vi "select_waveforms.vi"(0 "Trace controls":T6[](array[typedef]), 5 "Flag selectors":T4[](array[typedef]), 9 "Pose selectors":T1[](array[typedef]), 11 "Decimate":i32=1, 12 "Reference hold":bool) -> (4 "Waveforms out":waveform(sgl)[](array[waveform]), 6 "Digital waveforms":digitalwaveform[](array[waveform]), 8 "XY views":cluster{"X":sgl[], "Y":sgl[]}[](array[cluster]), 15 "New data":bool)   [LabVIEW 2013]
uses:
  Trace controls.ctl
  probe_point.ctl
  flag_selector.ctl
  status_flag.ctl
  pose_selector.ctl
  pose_source.ctl
  pose_relative_to.ctl
panel:
  out "Reference":sgl[][](array[numeric])
  out "Last waveforms out":waveform(sgl)[](array[waveform])
  in  "Old trace counter":u32
  # "Locals"
  # "Trace record that is the base for relative display"
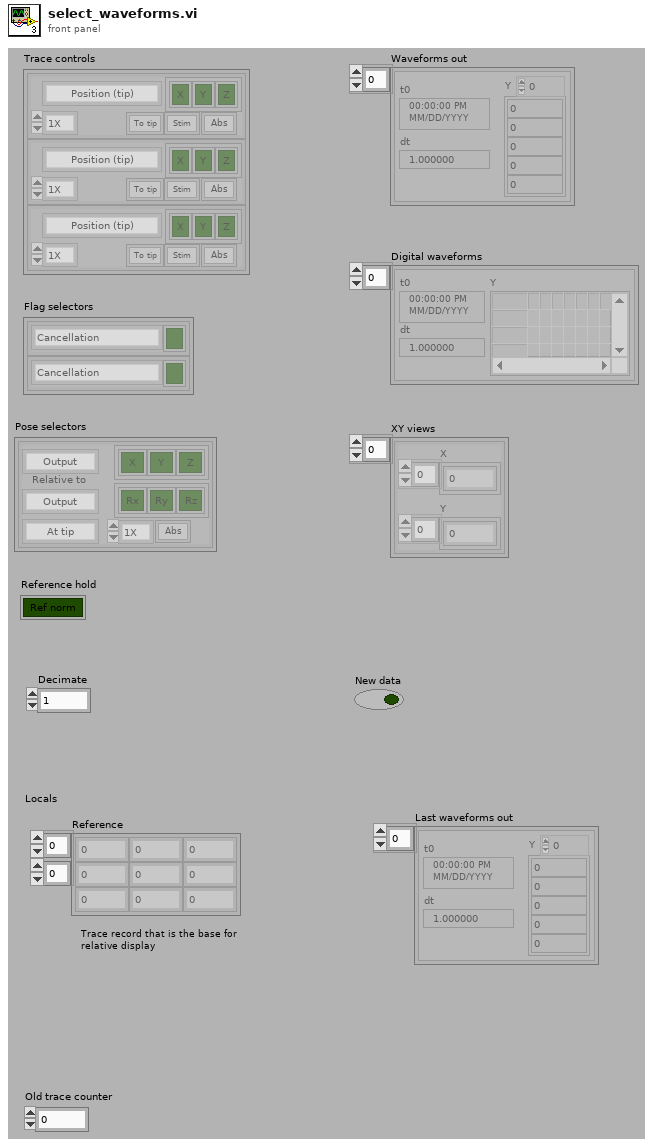
[diagram p1: front panel]
types:
  T1 = typedef "pose_selector.ctl" = cluster{"Scale":enum16{"1X", "10X", "100X", "1KX", "10KX"}, "Source":T2, "XYZ selector":cluster{"Boolean":bool, "Boolean 2":bool, "Boolean 3":bool}, "RPY selector":cluster{"Boolean":bool, "Boolean 2":bool, "Boolean 3":bool}, "Relative to":T3, "Relative":bool, "Translate":enum16{"At tip", "At RCM", "At KC", "At origin"}}
  T2 = typedef "pose_source.ctl" = enum16{"Output", "Handle", "Handle KF", "Goal", "Absolute"}
  T3 = typedef "pose_relative_to.ctl" = enum16{"Output", "Handle", "Handle KF", "Goal", "Absolute", "Trace start"}
  T4 = typedef "flag_selector.ctl" = cluster{"Flag":T5, "Select":bool}
  T5 = typedef "status_flag.ctl" = enum16{"Cancellation", "Goal filter", "Valid position", "Goal saturation tip", "Goal saturation RCM", "Goal circle saturation", "Position saturation", "Output saturation", "Acceleration limiting", "Finished late", "Stimulus increasing", "Integral error saturation", "Velocity limiting", "Log warning", "Log error", "Link KF degraded"}
  T6 = typedef "Trace controls.ctl" = cluster{"+ stim":bool, "Relative":bool, "Scale":enum16{"1X", "10X", "100X", "1KX", "10KX"}, "Probe point":T7, "XYZ selector":cluster{"Boolean":bool, "Boolean 2":bool, "Boolean 3":bool}, "To tip":bool}
  T7 = typedef "probe_point.ctl" = enum16{"Position (tip)", "Position (RCM)", "Null pos (tip)", "Null pos (RCM)", "V limiter (tip)", "V Limiter (RCM)", "Goal (tip)", "Goal (RCM)", "Link pos 0", "Link pos 1", "KF link pos 0", "KF link pos 1", "Link rate 0", "Link rate 1", "Link residue 0", "Link residue 1", "Link goal 0", "Link goal 1", "Rate limit 0", "Rate limit 1", "Link error 0", "Link error 1", "Controller 0", "Controller 1", "Output 0", "Output 1", "Drive 0", "Drive 1", "Stimulus 0", "Stimulus 1", "Trace data 0", "Trace data 1", "Analog data 0", "Analog data 1", "Status flags", "Light 0", "Light 1", "Light 2", "Light 3", "Light 4", "Light 5", "Goal origin", "Goal rotation 0", "Goal rotation 1", "Goal rotation 2", "Output origin", "Output rotation 0", "Output rotation 1", "Output rotation 2", "Handle origin", "Handle rotation 0", "Handle rotation 1", "Handle rotation 2", "Handle position", "Handle velocity", "Handle acceleration", "Handle angles", "Handle angle rates", "Handle pos residue", "Handle angle residue", "Trace length"}
  T8 = cluster{"Trace controls":T6[], "Flag selectors":T4[], "Decimate":i32, "Pose selectors":T1[], "Reference hold":bool}
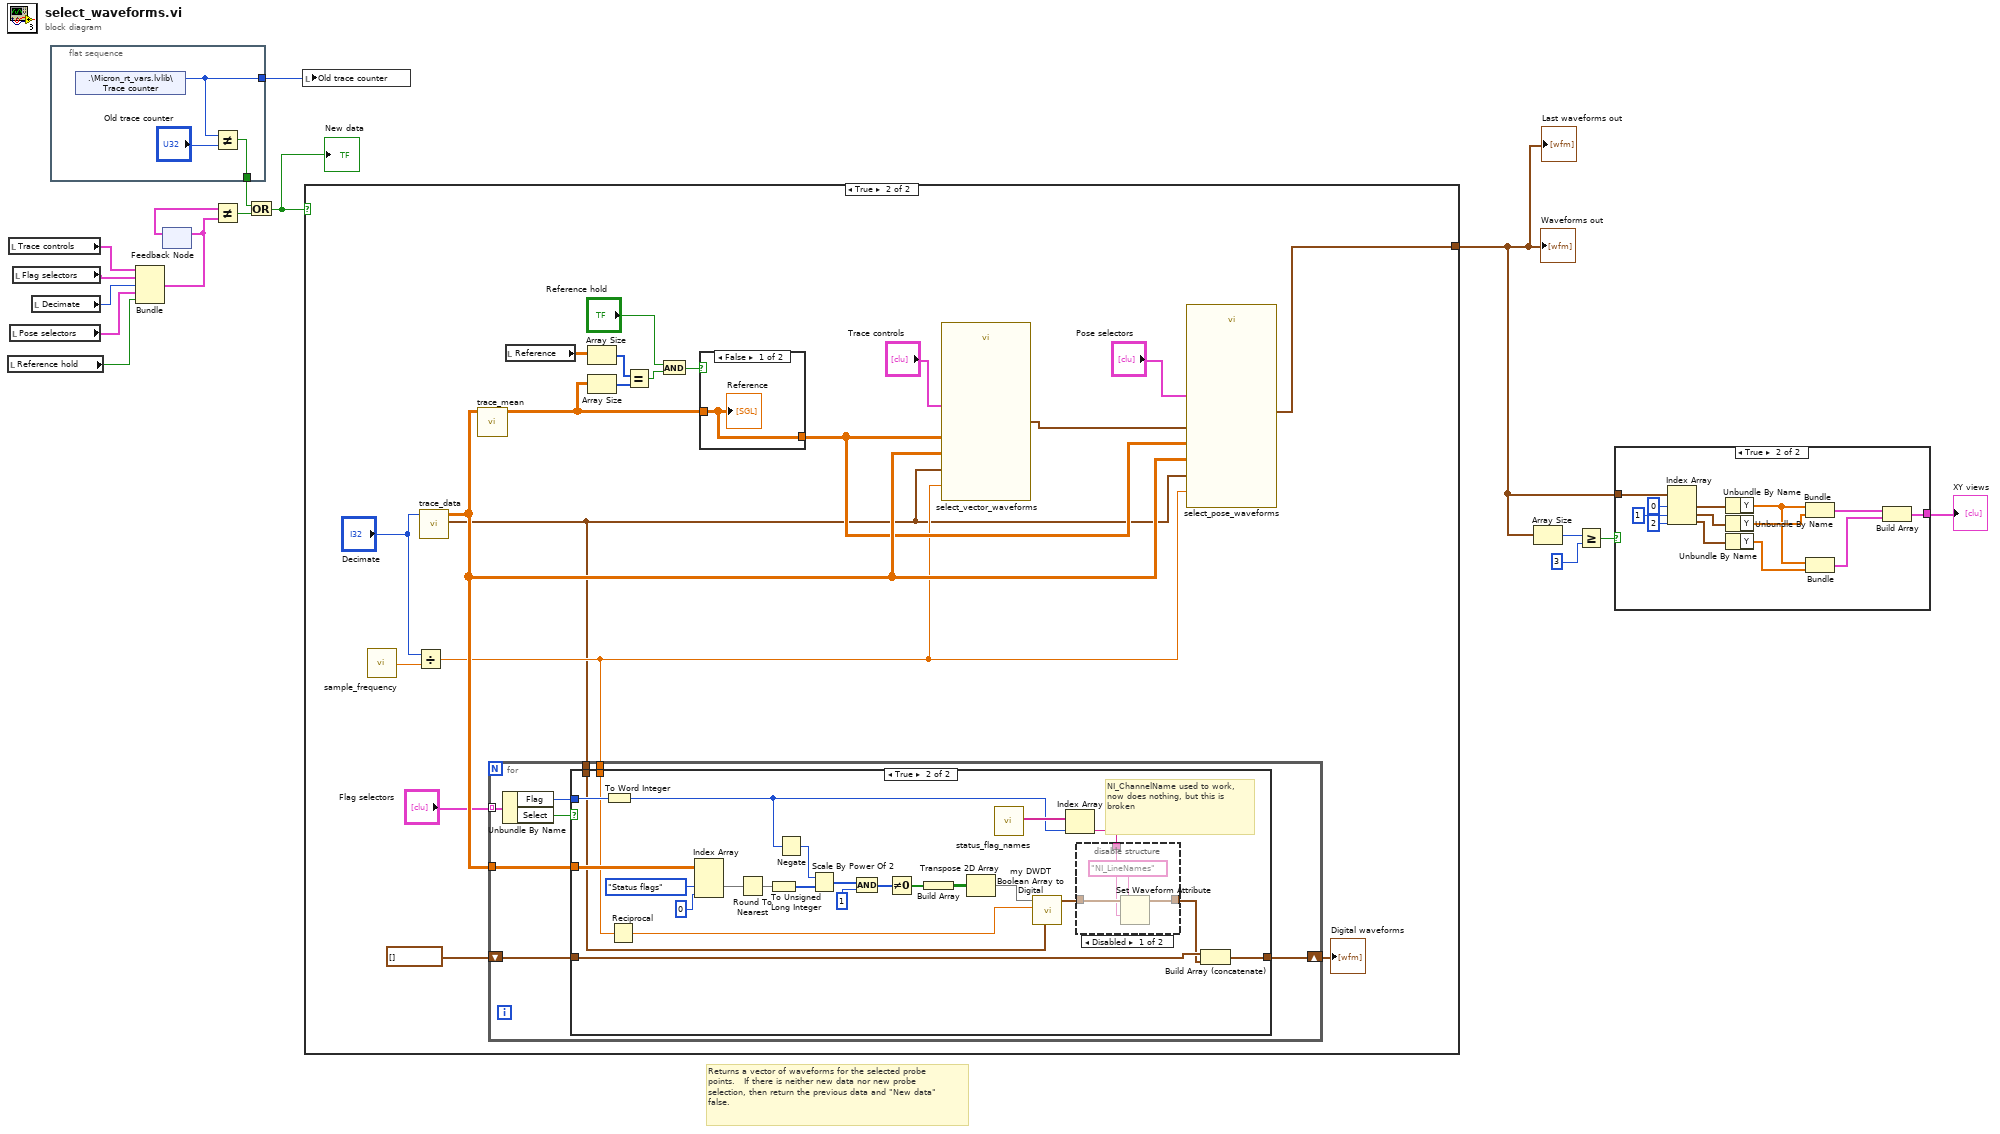
[diagram p0: block diagram]
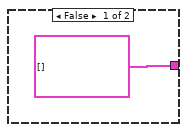
[diagram p2: hidden frame]
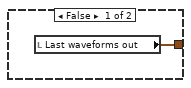
[diagram p3: hidden frame]
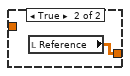
[diagram p4: hidden frame]
diagram:
  # "Returns a vector of waveforms for the selected probe points.   If there is neither new data nor new probe selection, then return the previous data and \"New data\" false."
  n1 = local read "Reference hold"() -> (w2:bool)
  n2 = local read "Trace controls"() -> (w8:T6[])
  n3 = local read "Pose selectors"() -> (w5:T1[])
  n4 = local read "Flag selectors"() -> (w7:T4[])
  n5 = local read "Decimate"() -> (w6:i32)
  n6 = flat-sequence {
    tunnel: [w18] -> w11
    tunnel: [w17] -> w16
    frame #0 {
      n7 = shared-variable ".\\Micron_rt_vars.lvlib\\Trace counter"() -> (w17:u32)  [unwired: 2 out]
      n8 = Not Equal?(x=w17, y="Old trace counter") -> (x != y?=w18:bool)
    }
  }
  n9 = Bundle("Trace controls"=w8, "Flag selectors"=w7, "Decimate"=w6, "Pose selectors"=w5, "Reference hold"=w2) -> (w4:T8)  [unwired: 1 in]
  n10 = feedback-in #1(w4) -> ()
  n11 = feedback #1() -> (w3:T8)  [unwired: 1 in]
  n12 = Not Equal?(x=w3, y=w4) -> (x != y?=w10:bool)
  n13 = Or(x=w11, y=w10) -> (x .or. y?=w9:bool)
  "New data" <- w9
  n14 = local write "Old trace counter"(w16) -> ()
  n15 = case shown="True" w9 {
    tunnel: [w20 w26] -> w1
    frame False {
      n16 = local read "Last waveforms out"() -> (w20:waveform(sgl)[])
    }
    frame True {
      n17 = call "sample_frequency.vi"() -> ("Sample frequency"=w39:dbl)
      n18 = Divide(x="Decimate", y=w39) -> (x/y=w23:dbl)
      n19 = call "trace_data.vi"("Decimate"="Decimate") -> ("Trace timestamp"=w21:timestamp, "Decimated trace"=w40:sgl[][][])  [unwired: 8 in, 1 out]
      n20 = call "trace_mean.vi"("Array in"=w40) -> ("Array out"=w22:sgl[][])  [unwired: 10 in]
      n21 = for {
        tunnel: "Flag selectors" -> [w50] mode=indexing
        tunnel: w40 -> [w48]
        shift-right: [w45] -> w35
        shift-left: digitalwaveform[] [] -> [w46]
        tunnel: w23 -> [w44]
        tunnel: w21 -> [w43]
        n22 = Unbundle By Name(w50) -> ("Flag"=w47:T5, "Select"=w49:bool)
        n23 = case shown="True" w49 {
          tunnel: w48 -> [_ w75]
          tunnel: w47 -> [_ w70]
          tunnel: w46 -> [w51 w64]
          tunnel: [w51 w60] -> w45
          tunnel: w44 -> [_ w62]
          tunnel: w43 -> [_ w53]
          frame False {
          }
          frame True {
            # "NI_ChannelName used to work, now does nothing, but this is broken"
            n24 = To Word Integer(number=w70) -> (16bit integer=w57:i16)
            n25 = Reciprocal(x=w62) -> (1/x=w61:dbl)
            n26 = Index Array(array=w75, index (dim 1)=probe_point."Status flags" ("Probe point"), index (dim 2)=0 ("disabled index (col)")) -> (element=w72:sgl[])  [unwired: 1 in]
            n27 = Round To Nearest(number=w72) -> (nearest integer value=w71:sgl[])
            n28 = To Unsigned Long Integer(number=w71) -> (unsigned 32bit integer=w68:u32[])
            n29 = Negate(x=w57) -> (-x=w69:i16)
            n30 = Scale By Power Of 2(n=w69, x=w68) -> (x*2^n=w67:u32[])
            n31 = And(x=w67, y=u32 1 ("disabled index (col)")) -> (x .and. y?=w65:u32[])
            n32 = Not Equal To 0?(x=w65) -> (x != 0?=w63:bool[])
            n33 = Build Array(w63) -> (w55:bool[][])
            n34 = Transpose 2D Array(2D array=w55) -> (transposed array=w54:bool[][])
            n35 = call "status_flag_names.vi"() -> ("Names"=w58:string[])  [unwired: 11 in]
            n36 = call "my DWDT Boolean Array to Digital.vi"("t0"=w53, "sample rate"=w61, "boolean array"=w54) -> ("digital waveform"=w59:digitalwaveform)  [unwired: 7 in, 1 out]
            n37 = Index Array(array=w58, index=w57) -> (element=w56:string)
            n38 = disable-structure shown="Disabled" {
              disable-tunnel: w59 -> [w78 w80]
              disable-tunnel: w56 -> [w77 _]
              disable-tunnel: [w76 w80] -> w52
              frame Disabled {
                n39 = Set Waveform Attribute(5:w77, 6:"NI_LineNames" ("name"), 7:w78) -> (3:w76:digitalwaveform)  [unwired: 1 in, 2 out]
              }
              frame Enabled {
              }
            }
            n40 = Build Array (concatenate)(w64, w52) -> (w60:digitalwaveform[])
          }
        }
      }
      "Digital waveforms" <- w35
      n41 = local read "Reference"() -> (w33:sgl[][])
      n42 = Array Size(array=w33) -> (size(s)=w32:i32[])
      n43 = Array Size(array=w22) -> (size(s)=w31:i32[])
      n44 = Equal?(x=w32, y=w31) -> (x = y?=w30:bool)
      n45 = And(x="Reference hold", y=w30) -> (x .and. y?=w28:bool)
      n46 = case shown="False" w28 {
        tunnel: w22 -> [w41 _]
        tunnel: [w41 w42] -> w24
        frame False {
          "Reference" <- w41
        }
        frame True {
          n47 = local read "Reference"() -> (w42:sgl[][])
        }
      }
      n48 = call "select_vector_waveforms.vi"("Trace timestamp"=w21, "Decimated dt"=w23, "Decimated trace"=w40, "Reference"=w24, "Trace controls"="Trace controls") -> ("Waveforms out"=w27:waveform(sgl)[])  [unwired: 6 in]
      n49 = call "select_pose_waveforms.vi"("Trace timestamp"=w21, "Decimated trace"=w40, "Decimated dt"=w23, "Reference"=w24, "Pose selectors"="Pose selectors", "Waveforms in"=w27) -> ("Waveforms out"=w26:waveform(sgl)[])  [unwired: 5 in]
    }
  }
  "Waveforms out" <- w1
  "Last waveforms out" <- w1
  n50 = Array Size(array=w1) -> (size(s)=w15:i32)
  n51 = Greater Or Equal?(x=w15, y=3) -> (x >= y?=w13:bool)
  n52 = case shown="True" w13 {
    tunnel: w1 -> [_ w94]
    tunnel: [cluster{"Y":sgl[], "Y":sgl[]}[] [] w85] -> w12
    frame False {
    }
    frame True {
      n53 = Index Array(array=w94, index #1=0 ("index"), index #2=1 ("index"), index #3=2 ("index")) -> (element #1=w90:waveform(sgl), element #2=w89:waveform(sgl), element #3=w88:waveform(sgl))
      n54 = Unbundle By Name(w90) -> ("Y"=w83:sgl[])
      n55 = Unbundle By Name(w89) -> ("Y"=w84:sgl[])
      n56 = Unbundle By Name(w88) -> ("Y"=w82:sgl[])
      n57 = Bundle("Y"=w83, "Y"=w84) -> (w87:cluster{"Y":sgl[], "Y":sgl[]})  [unwired: 1 out]
      n58 = Bundle("Y"=w83, "Y"=w82) -> (w86:cluster{"Y":sgl[], "Y":sgl[]})  [unwired: 1 out]
      n59 = Build Array(w87, w86) -> (w85:cluster{"Y":sgl[], "Y":sgl[]}[])
    }
  }
  "XY views" <- w12
